vi "DiscArchiver.constructor.vi"(0 "name":string, 2 "data in":string, 5 "error in (no error)":errorcluster) -> (14 "i ref out":refnum<vi>, 16 "data out":string, 19 "error out":errorcluster)   [LabVIEW 2014, in "DiscArchiver.lvlib"]
doc: "Gets data from a data collector and writes it to disk. The DiscArchiver is initialized by the \"RegisterToCollector\" method. It obtains descriptionData of a run and the eventData of a run via DIM services\n\nLicense Agreement for this software:\n\nCopyright (C)\nGesellschaft für Schwerionenforschung, GSI\nPlanckstr. 1\n64291 Darmstadt\nGermany\n\nContact: D.Beck@gsi.de \n\nThis program is free software; you can redistribute it and/or modify it under the terms of the \nGNU General Public License as published by the Free Software Foundation; either version 2 of \nthe license, or (at your option) any later version.\n\nThis program is distributed in the hope that it will be useful, but WITHOUT ANY WARRANTY; \nwithout even the implied warranty of MERCHANTABILITY or FITNESS FOR A PARTICULAR PURPOSE. See the GNU General License for more details (http://www.gnu.org).\n\nGesellschaft für Schwerionenforschung, GSI\nPlanckstr. 1, 64291 Darmstadt, Germany\nFor all questions and ideas contact: M.Richter@gsi.de, H.Brand@gsi.de or D.Beck@gsi.de.\nLast update: 16-JUN-2004"
uses:
  DiscArchiver.lvlib
  CSCore/BaseProcess/BaseProcess.lvlib
  CSCore/CSSystem/CSSystemLib/CSSystemLib.lvlib
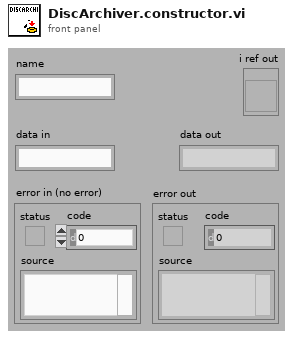
[diagram p1: front panel]
types:
  T1 = enum16{"SetAttribute", "GetAttribute", "CreateAttribute", "DestroyAttribute", "DestroyAllAtributes"}
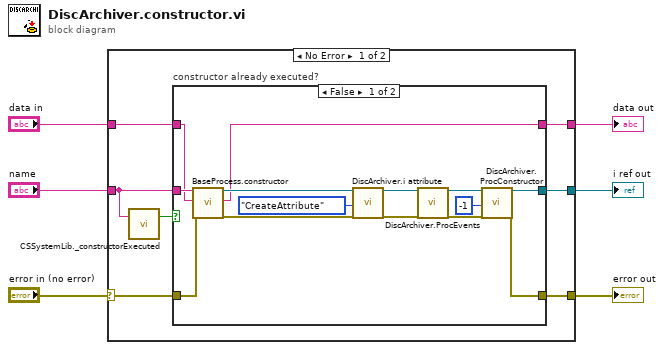
[diagram p0: block diagram]
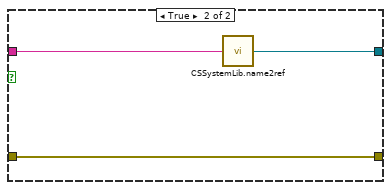
[diagram p2: hidden frame]
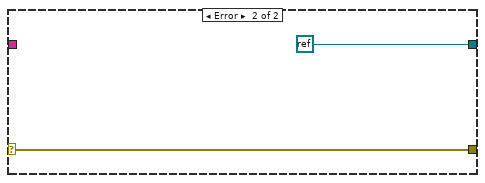
[diagram p3: hidden frame]
diagram:
  n1 = case shown="No Error" "error in (no error)" {
    selector: "error in (no error)" -> [w11 w31]
    tunnel: "name" -> [w9 _]
    tunnel: [w13 refnum<k0> refnum] -> w5
    tunnel: [w12 w31] -> w4
    tunnel: "data in" -> [w8 _]
    tunnel: [w7 _] -> w1
    frame No Error {
      n2 = call "CSSystemLib._constructorExecuted.vi"("name"=w9) -> ("constructor executed?"=w10:bool)  [unwired: 18 in]
      n3 = case "constructor already executed?" shown="False" w10 {
        tunnel: w9 -> [w24 w30]
        tunnel: [w18 w29] -> w13
        tunnel: [w17 w28] -> w12
        tunnel: w11 -> [w16 w28]
        tunnel: w8 -> [w15 _]
        tunnel: [w14 _] -> w7
        frame False {
          n4 = call "BaseProcess.constructor.vi"("name"=w24, "data in"=w15, "error in (no error)"=w16) -> ("i ref out"=w27:refnum<vi>, "data out"=w14:string, "error out"=w26:errorcluster)  [unwired: 14 in]
          n5 = call "DiscArchiver.i attribute.vi"("VI Refnum"=w27, "Action"=T1."CreateAttribute", "error in (no error)"=w26) -> ("VI Refnum out"=w23:refnum<vi>, "error out"=w22:errorcluster)  [unwired: 14 in, 1 out]
          n6 = call "DiscArchiver.ProcEvents.vi"("i ref in"=w23, "error in (no error)"=w22) -> ("i ref out"=w21:refnum<vi>, "error out"=w20:errorcluster)  [unwired: 16 in]
          n7 = call "DiscArchiver.ProcConstructor.vi"("i ref in"=w21, "ms timeout (10000)"=-1 ("ms timeout (100)"), "error in (no error)"=w20) -> ("i ref out"=w18:refnum<vi>, "error out"=w17:errorcluster)  [unwired: 14 in, 1 out]
        }
        frame True {
          n8 = call "CSSystemLib.name2ref.vi"("name"=w30) -> ("obj refnum"=w29:refnum<vi>)
        }
      }
    }
    frame Error {
    }
  }
  "i ref out" <- w5
  "error out" <- w4
  "data out" <- w1
